vi "subPos.vi"(1 "POS":cluster{"X":dbl, "Y":dbl, "Z":dbl}, 2 "NewVal":cluster{"X":sgl, "Y":sgl, "Z":sgl}) -> (0 "PosSetG92":cluster{"X":dbl, "Y":dbl, "Z":dbl})   [LabVIEW 2017]
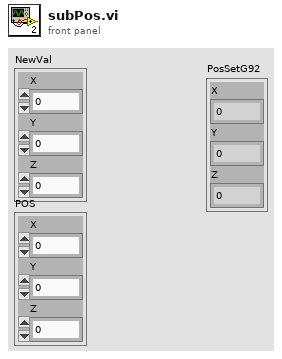
[diagram p1: front panel]
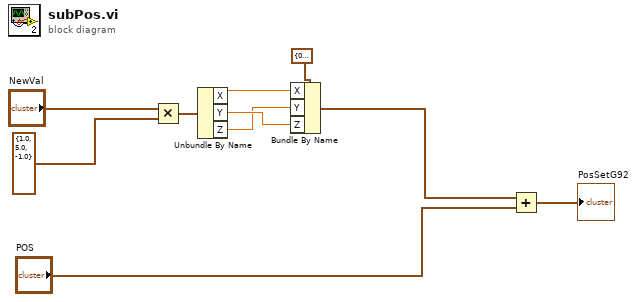
[diagram p0: block diagram]
diagram:
  n1 = Multiply(x="NewVal", y=cluster{"X":dbl, "Y":dbl, "Z":dbl} {"X"=1.0, "Y"=5.0, "Z"=-1.0} ("PosSetG92")) -> (x*y=w8:cluster{"X":dbl, "Y":dbl, "Z":dbl})
  n2 = Unbundle By Name(w8) -> ("X"=w6:dbl, "Y"=w5:dbl, "Z"=w4:dbl)
  n3 = Bundle By Name(cluster=cluster{"X":dbl, "Y":dbl, "Z":dbl} {"X"=0.0, "Y"=0.0, "Z"=0.0} ("PosSetG92"), "X"=w6, "Y"=w4, "Z"=w5) -> (w1:cluster{"X":dbl, "Y":dbl, "Z":dbl})
  n4 = Add(x=w1, y="POS") -> (x+y=→"PosSetG92":cluster{"X":dbl, "Y":dbl, "Z":dbl})
